vi "ReadResults.vi"(11 "VISA resource":refnum<visa-resource-name>) -> (0 "error out":errorcluster, 2 "Energy/Power(SI)":dbl[](array[numeric]))   [LabVIEW 2012]
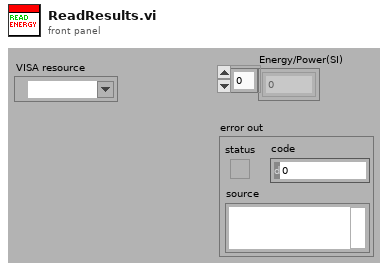
[diagram p1: front panel]
types:
  T1 = enum16{"Initialize", "Write", "Write/Read", "Read", "Clear", "Close"}
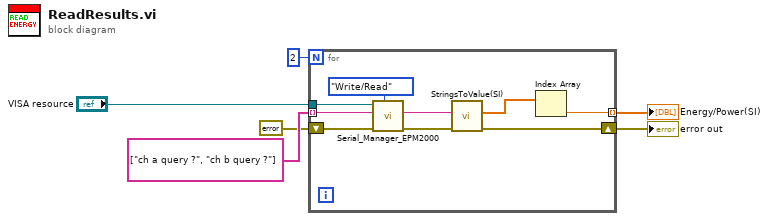
[diagram p0: block diagram]
diagram:
  n1 = for {
    N: 2 -> [_]
    tunnel: "VISA resource" -> [w14]
    tunnel: string[] ["ch a query ?", "ch b query ?"] -> [w12] mode=indexing
    shift-right: [w9] -> w5
    shift-left: errorcluster {"status"=FALSE, "code"=0, "source"=""} ("error out") -> [w13]
    tunnel: [w8] -> w2 mode=indexing
    n2 = call "Serial_Manager_EPM2000.vi"("Job"=T1."Write/Read", "error in"=w13, "write buffer"=w12, "VISA resource"=w14) -> ("error out"=w10:errorcluster, "read buffer"=w11:string)  [unwired: 6 in]
    n3 = call "StringsToValue(SI).vi"("error in"=w10, "input string"=w11) -> ("error out"=w9:errorcluster, "Energy/Power(SI)"=w7:dbl[])  [unwired: 8 in]
    n4 = Index Array(array=w7) -> (element=w8:dbl)  [unwired: 1 in]
  }
  "error out" <- w5
  "Energy/Power(SI)" <- w2
